vi "cal avg rate.vi"(8 "error in (no error)":errorcluster, 11 "Automation in":refnum<class "Automation.lvclass">) -> (0 "error out":errorcluster, 2 "Average rate":dbl, 3 "Automation out":refnum<class "Automation.lvclass">)   [LabVIEW 2019, in "Automation.lvclass"]
uses:
  Automation.lvclass
  Automation.lvclass/Automation.ctl
  <vilib>/Analysis/baseanly.llb/Mean (DBL).vi
  <vilib>/Analysis/NI_AALBase.lvlib
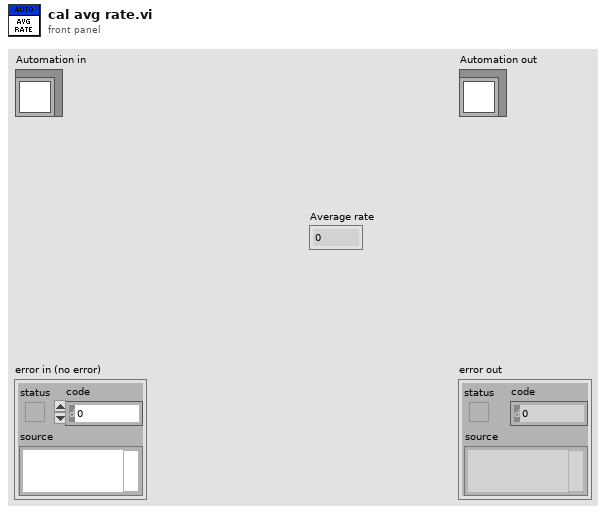
[diagram p1: front panel]
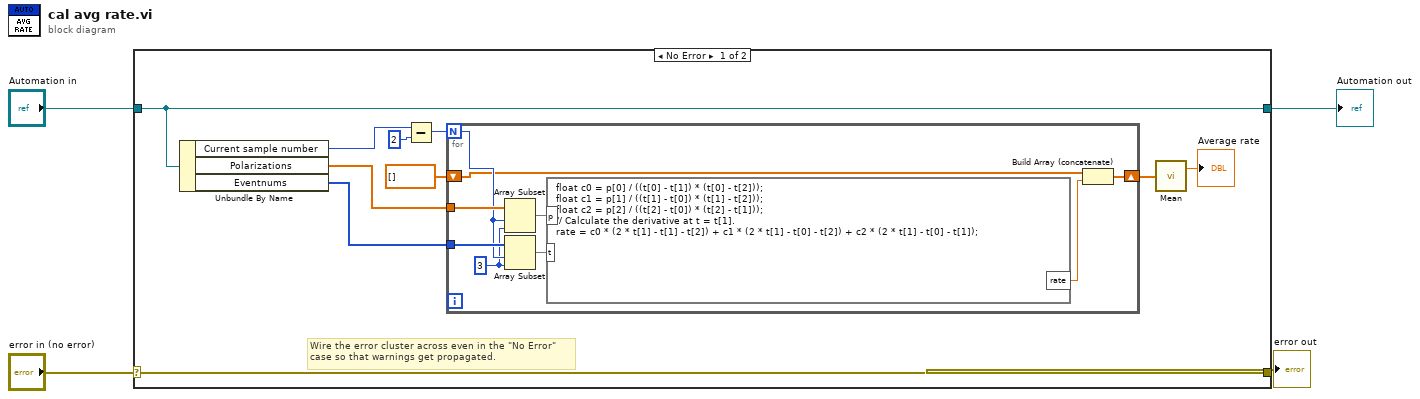
[diagram p0: block diagram]
diagram:
  n1 = case shown="No Error" "error in (no error)" {
    selector: "error in (no error)" -> [w14 w25]
    tunnel: [w14 w25] -> w3
    tunnel: [w13 w24] -> w1
    tunnel: "Automation in" -> [w13 w24]
    frame No Error {
      # "Wire the error cluster across even in the \"No Error\"\ncase so that warnings get propagated."
      n2 = Unbundle By Name(w13) -> ("Current sample number"=w5:i32, "Polarizations"=w6:dbl[], "Eventnums"=w7:i64[])
      n3 = Subtract(x=w5, y=2) -> (x-y=w10:i32)
      n4 = for {
        N: w10 -> [w21]
        shift-right: [w16] -> w8
        shift-left: dbl[] [] -> [w18]
        tunnel: w6 -> [w23]
        tunnel: w7 -> [w22]
        w20 = 3 ("length")
        n5 = Array Subset(array=w23, index=w21, length=w20) -> (w15:dbl[])
        n6 = Array Subset(array=w22, index=w21, length=w20) -> (w19:i64[])
        n7 = formula code="float c0 = p[0] / ((t[0] - t[1]) * (t[0] - t[2]));\nfloat c1 = p[1] / ((t[1] - t[0]) * (t[1] - t[2]));\nfloat c2 = p[2] / ((t[2] - t[0]) * (t[2] - t[1]));\n// Calculate the derivative at t = t[1].\nrate = c0 * (2 * t[1] - t[1] - t[2]) + c1 * (2 * t[1] - t[0] - t[2]) + c2 * (2 * t[1] - t[0] - t[1]);"("p"=w15, "t"=w19) -> ("rate"=w17:dbl)
        n8 = Build Array (concatenate)(w18, w17) -> (w16:dbl[])
      }
      n9 = call-poly <vilib>:"Mean.vi"("X"=w8) -> ("mean"=→"Average rate":dbl)  [unwired: 1 out]
    }
    frame Error {
    }
  }
  "error out" <- w3
  "Automation out" <- w1
